vi "Configure Self-Test.vi"(6 "Enable V0 self- test (T: Enable)":bool=TRUE, 7 "Enable VCOM self- test (T: Enable)":bool=TRUE, 8 "error in (no error)":errorcluster, 9 "Enable VRF Self-test (T: Enable)":bool=TRUE, 10 "Enable Reference Calibrator Self-test (T: Enable)":bool=TRUE, 11 "VISA resource name":refnum<visa-resource-name>) -> (0 "error out":errorcluster, 3 "VISA resource name out":refnum<visa-resource-name>)   [LabVIEW 2011, in "Agilent N432A.lvlib"]
doc: "Enables or disables several procedure of self-test during power up. It can be used while the self- test incorrectly indicates a failure."
uses:
  <instrlib>/Agilent N432A/Agilent N432A.lvlib
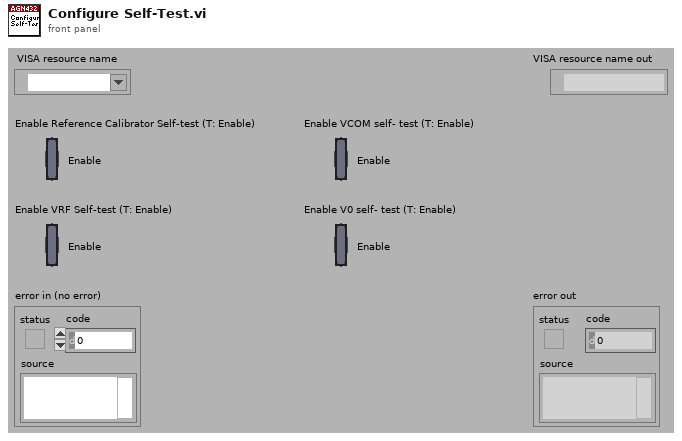
[diagram p1: front panel]
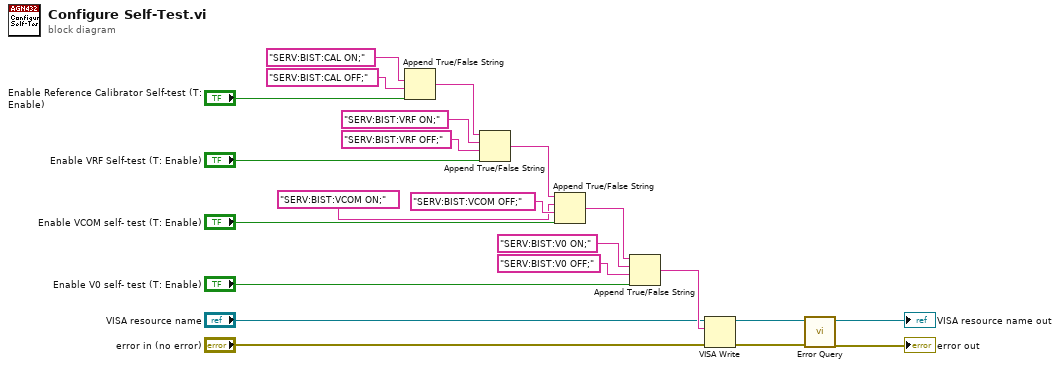
[diagram p0: block diagram]
diagram:
  n1 = Append True/False String(1:"Enable Reference Calibrator Self-test (T: Enable)", 2:"SERV:BIST:CAL OFF;", 3:"SERV:BIST:CAL ON;") -> (0:w19:string)  [unwired: 1 in]
  n2 = Append True/False String(1:"Enable VRF Self-test (T: Enable)", 2:"SERV:BIST:VRF OFF;", 3:"SERV:BIST:VRF ON;", 4:w19) -> (0:w15:string)
  n3 = Append True/False String(1:"Enable VCOM self- test (T: Enable)", 2:"SERV:BIST:VCOM OFF;", 3:"SERV:BIST:VCOM ON;", 4:w15) -> (0:w11:string)
  n4 = Append True/False String(1:"Enable V0 self- test (T: Enable)", 2:"SERV:BIST:V0 OFF;", 3:"SERV:BIST:V0 ON;", 4:w11) -> (0:w7:string)
  n5 = VISA Write(VISA resource name="VISA resource name", write buffer=w7, error in (no error)="error in (no error)") -> (VISA resource name out=w4:refnum<visa-resource-name>, error out=w3:errorcluster)  [unwired: 1 out]
  n6 = call <instrlib>:"Error Query.vi"("error in (no error)"=w3, "VISA resource name"=w4) -> ("error out"=→"error out":errorcluster, "VISA resource name out"=→"VISA resource name out":refnum<visa-resource-name>)  [unwired: 6 in, 2 out]
